vi "Log Wait Motion Helper.vi"(4 "MaxCntExceeded":bool, 5 "Timeout":i32, 6 "Cancel":bool, 7 "State Info":string, 8 "error in (no error)":errorcluster, 9 "Status":u16, 10 "Loop Count":i32, 11 "EventLog in":refnum<class "EventLog.lvclass">) -> (0 "error out":errorcluster, 3 "EventLog out":refnum<class "EventLog.lvclass">)   [LabVIEW 2015, in "Tool Module.lvlib"]
uses:
  Tool Module.lvlib
  Event Logger Library/Event Log/EventLog.lvclass
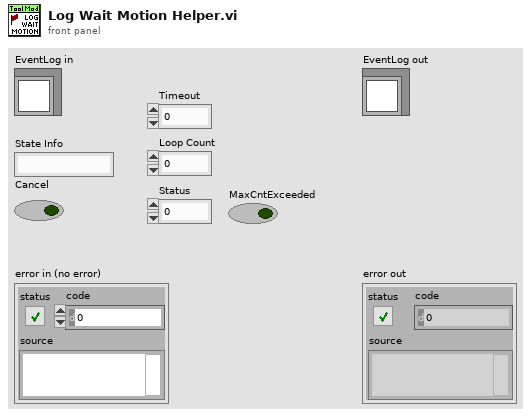
[diagram p1: front panel]
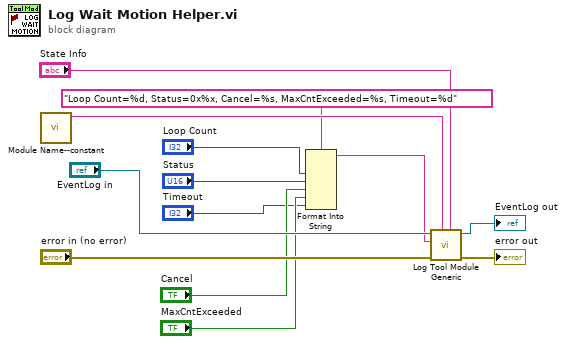
[diagram p0: block diagram]
diagram:
  n1 = call "Module Name--constant.vi"() -> ("Module Name"=w13:string)  [unwired: 11 in]
  n2 = Format Into String(format string="Loop Count=%d, Status=0x%x, Cancel=%s, MaxCntExceeded=%s, Timeout=%d", "Loop Count", "Status", "Cancel", "MaxCntExceeded", "Timeout") -> (resulting string=w4:string)  [unwired: 2 in, 1 out]
  n3 = call "Log Tool Module Generic.vi"("State Info"="State Info", "Module Name"=w13, "error in (no error)"="error in (no error)", "Payload"=w4, "EventLog in"="EventLog in") -> ("error out"=→"error out":errorcluster, "EventLog out"=→"EventLog out":refnum<class "EventLog.lvclass">)  [unwired: 5 in]
